vi "sequence4Digit.vi"(8 "Error In":errorcluster, 11 "Trace Number In":string) -> (0 "Error Out":errorcluster, 3 "Trace Number Out":string)   [LabVIEW 2018]
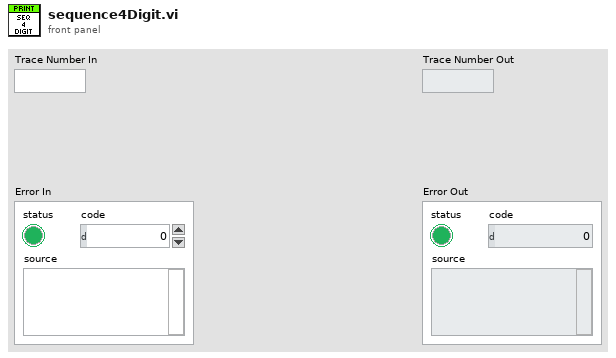
[diagram p1: front panel]
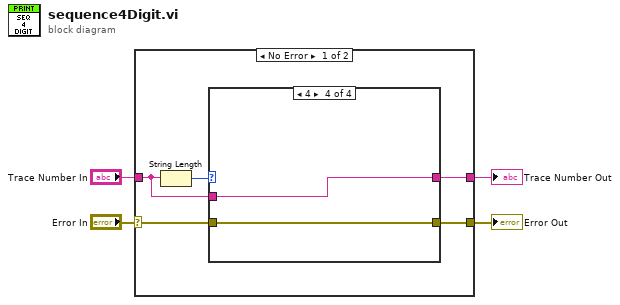
[diagram p0: block diagram]
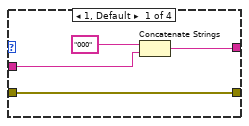
[diagram p2: hidden frame]
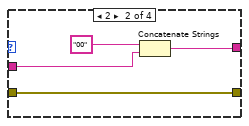
[diagram p3: hidden frame]
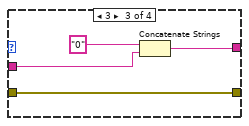
[diagram p4: hidden frame]
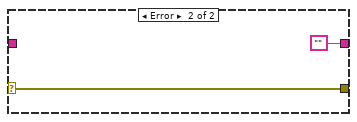
[diagram p5: hidden frame]
diagram:
  n1 = case shown="No Error" "Error In" {
    selector: "Error In" -> [w9 w25]
    tunnel: [w8 w25] -> w3
    tunnel: "Trace Number In" -> [w6 _]
    tunnel: [w5 ""] -> w1
    frame No Error {
      n2 = String Length(string=w6) -> (length=w7:i32)
      n3 = case shown="4" w7 {
        tunnel: w9 -> [w13 w17 w21 w23]
        tunnel: [w13 w17 w21 w23] -> w8
        tunnel: w6 -> [w11 w15 w19 w22]
        tunnel: [w10 w14 w18 w22] -> w5
        frame 1, Default {
          n4 = Concatenate Strings("000", w11) -> (w10:string)
        }
        frame 2 {
          n5 = Concatenate Strings("00", w15) -> (w14:string)
        }
        frame 3 {
          n6 = Concatenate Strings("0", w19) -> (w18:string)
        }
        frame 4 {
        }
      }
    }
    frame Error {
    }
  }
  "Trace Number Out" <- w1
  "Error Out" <- w3
